vi "GlobalSavePathToStoreStack.vi"() -> ()   [LabVIEW 2010]
panel:
  in  "SaveStackPath":path
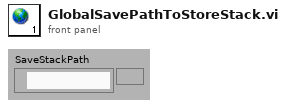
[diagram p1: front panel]
diagram:
